vi "RT_Test_auto set time.vi"() -> ()   [LabVIEW 2018]
uses:
  PublicSubVI/Ctl/_ctl_RT_D999_Command.ctl
panel:
  out "error out":errorcluster
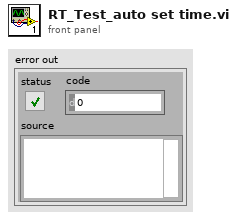
[diagram p1: front panel]
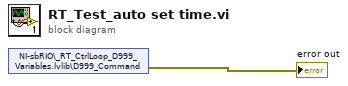
[diagram p0: block diagram]
diagram:
  n1 = shared-variable "NI-sbRIO\\_RT_CtrlLoop_D999_Variables.lvlib\\D999_Command"() -> (error out=→"error out":errorcluster)  [unwired: 1 in, 1 out]
